vi "calibration.vi"() -> ()   [LabVIEW 2012]
uses:
  globalstatus.vi
  globalreport.vi
  globalsettings.vi
panel:
  in  "in sn 3":string
  in  "status":u16(ring) items=["idle", "read sn", "write sn", "adjust dac", "collect", "write coefficient", "check do"]
  in  "in sn 7":string
  out "working 7":bool
  out "sn 7":string
  in  "port 7":refnum<visa-resource-name>
  in  "in sn 6":string
  out "working 6":bool
  out "sn 6":string
  in  "port 6":refnum<visa-resource-name>
  in  "in sn 5":string
  out "working 5":bool
  out "sn 5":string
  in  "port 5":refnum<visa-resource-name>
  in  "in sn 4":string
  out "working 4":bool
  out "sn 4":string
  in  "port 4":refnum<visa-resource-name>
  out "working 3":bool
  out "sn 3":string
  in  "port 3":refnum<visa-resource-name>
  in  "in sn 2":string
  in  "in sn 1":string
  out "working 2":bool
  out "working 1":bool
  out "working":bool
  out "sn 2":string
  out "sn 1":string
  out "sn":string
  in  "run":bool
  in  "golden port":refnum<visa-resource-name>
  in  "port 2":refnum<visa-resource-name>
  in  "port 1":refnum<visa-resource-name>
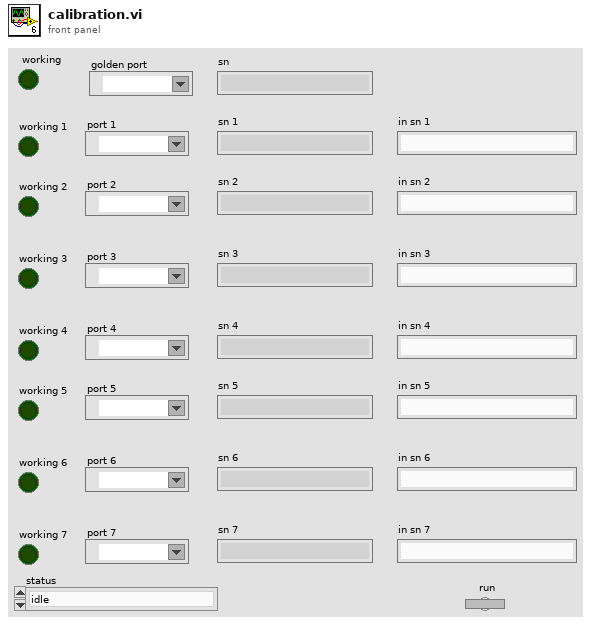
[diagram p1: front panel]
types:
  T1 = cluster{"B0":dbl, "B1":dbl, "K":dbl, "B":dbl, "B2":dbl}
  T2 = cluster{"port 7":refnum<visa-resource-name>, string, dbl, dbl, dbl, dbl, dbl, dbl, dbl, dbl, dbl, dbl, dbl, dbl, dbl, dbl, dbl, "B0":dbl, "B1":dbl, "B2":dbl, "K":dbl, "B":dbl, string, string}
  T3 = cluster{"Ten 0%":dbl, "Ten 5%":dbl, "Ten 10%":dbl, "Ten 20%":dbl, "Tolerance":dbl, "Ten 15%":dbl, "Ten 40%":dbl, "Ten 100%":dbl, "Times":dbl}
  T4 = cluster{"PORT":string, "SN":string, "RED DAC":dbl, "BLUE DAC":dbl, "RED AMP":dbl, "BLUE AMP":dbl, "T0":dbl, "T1":dbl, "T2":dbl, "T3":dbl, "T4":dbl, "T5":dbl, "T6":dbl, "A0":dbl, "A1":dbl, "A2":dbl, "A3":dbl, "B0":dbl, "B1":dbl, "B2":dbl, "C1":dbl, "C0":dbl, "result":string, "error":string}[]
  T5 = cluster{"port 7":refnum<visa-resource-name>, string, string, string, string, string, string, string, string, string, string}
  T6 = cluster{"DO 0%":dbl, "DO 5%":dbl, "DO 10%":dbl, "DO 20%":dbl, "Tolerance":dbl, "DO 15%":dbl, "DO 40%":dbl, "DO 100%":dbl, "Times":dbl}
  T7 = cluster{"PORT":string, "SN":string, "DO 0":string, "DO 1":string, "DO 2":string, "DO 3":string, "DO 4":string, "DO 5":string, "DO 6":string, "result":string, "error":string}[]
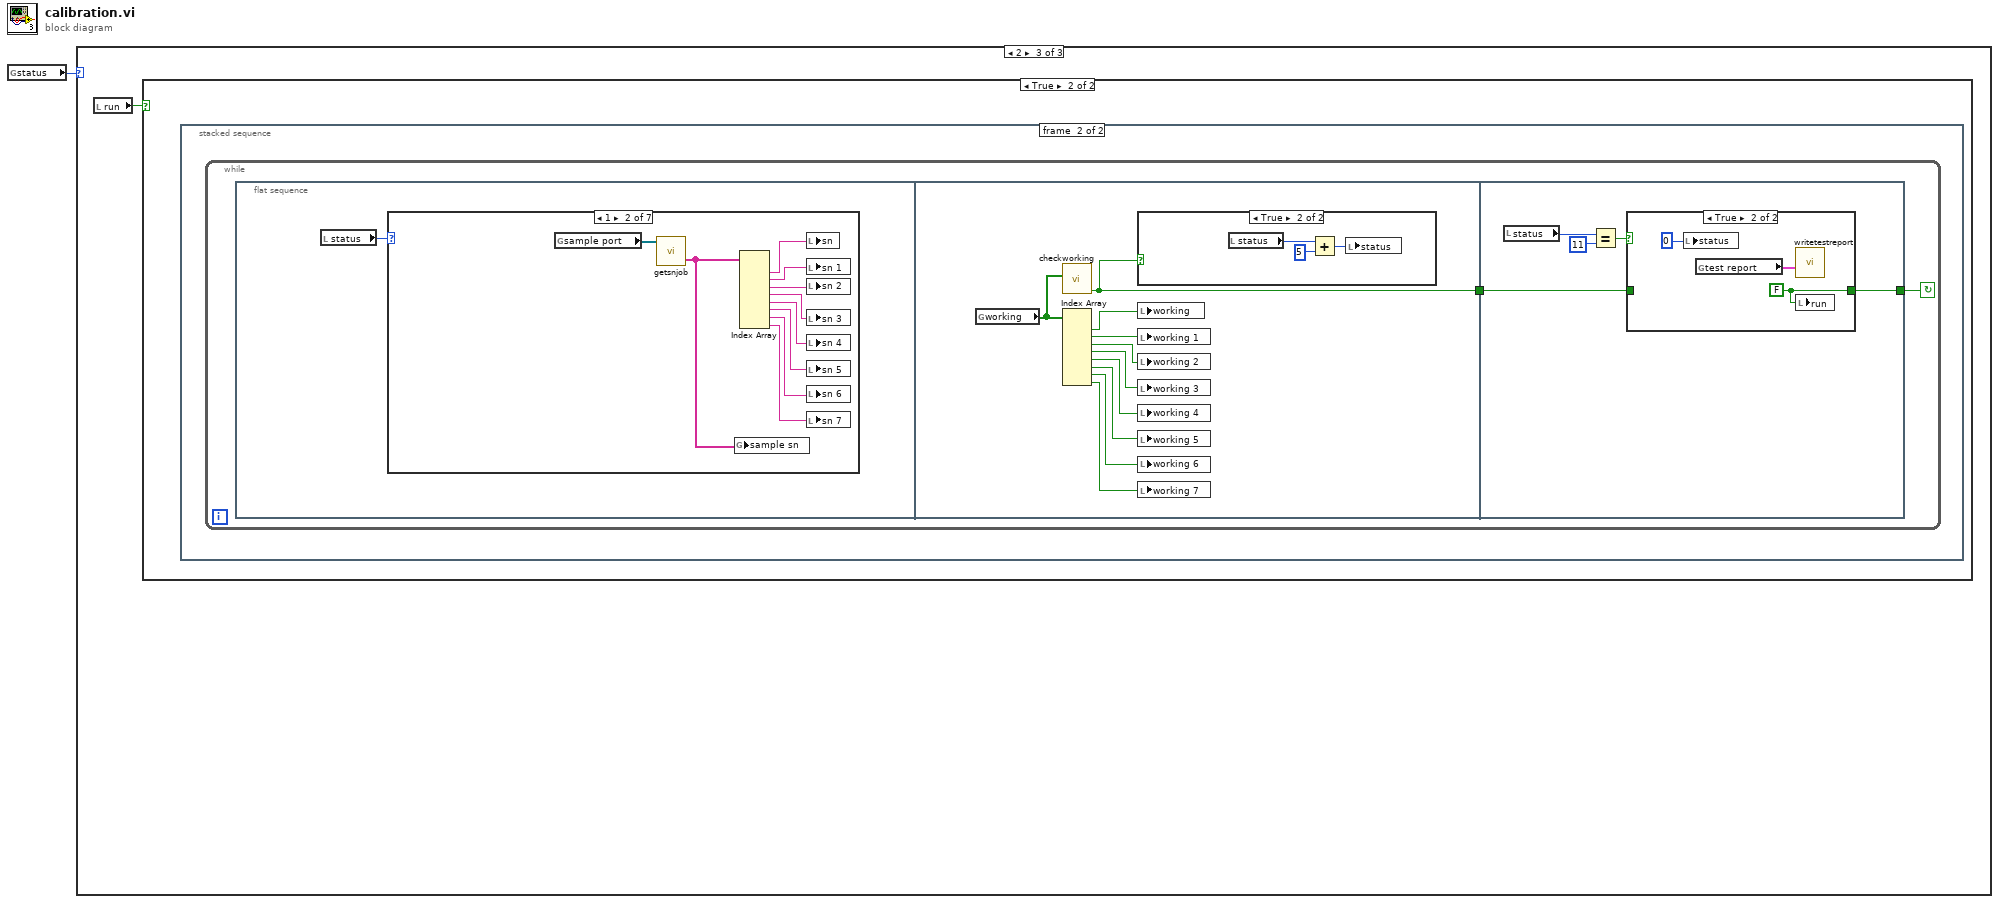
[diagram p0: block diagram]
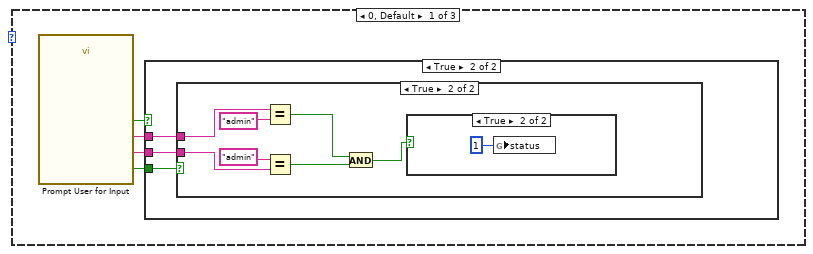
[diagram p2: hidden frame]
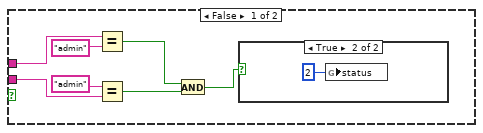
[diagram p4: hidden frame]
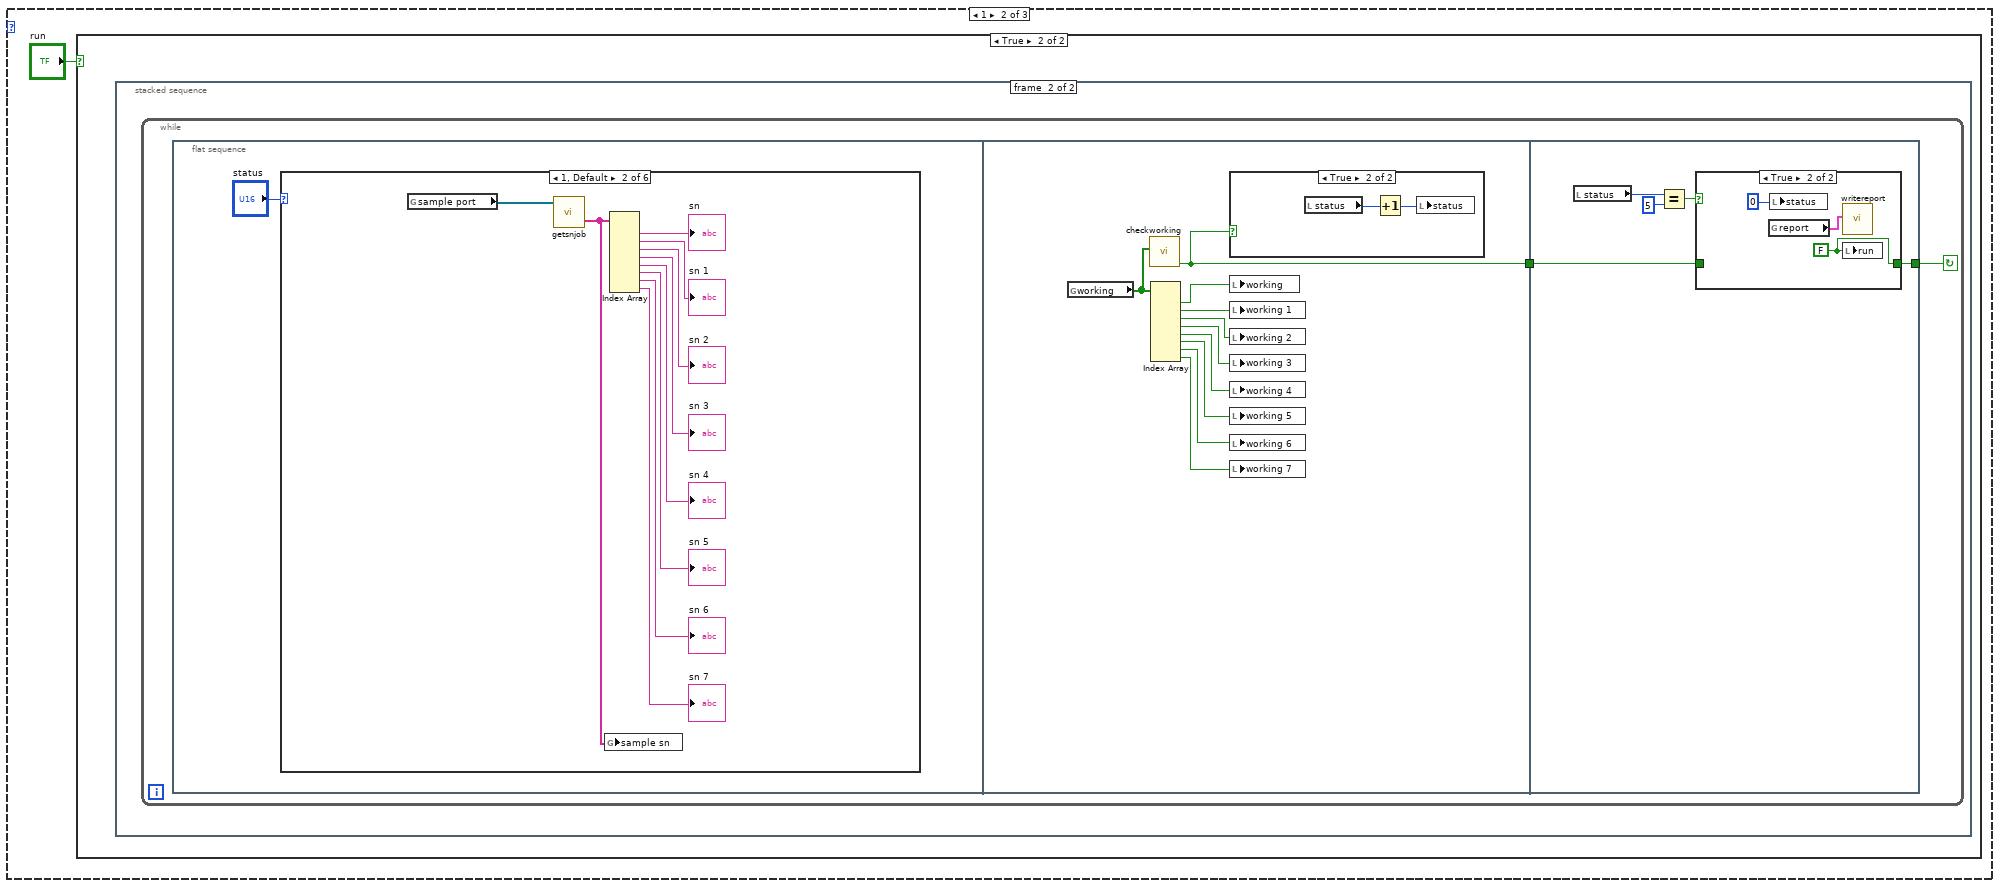
[diagram p7: hidden frame]
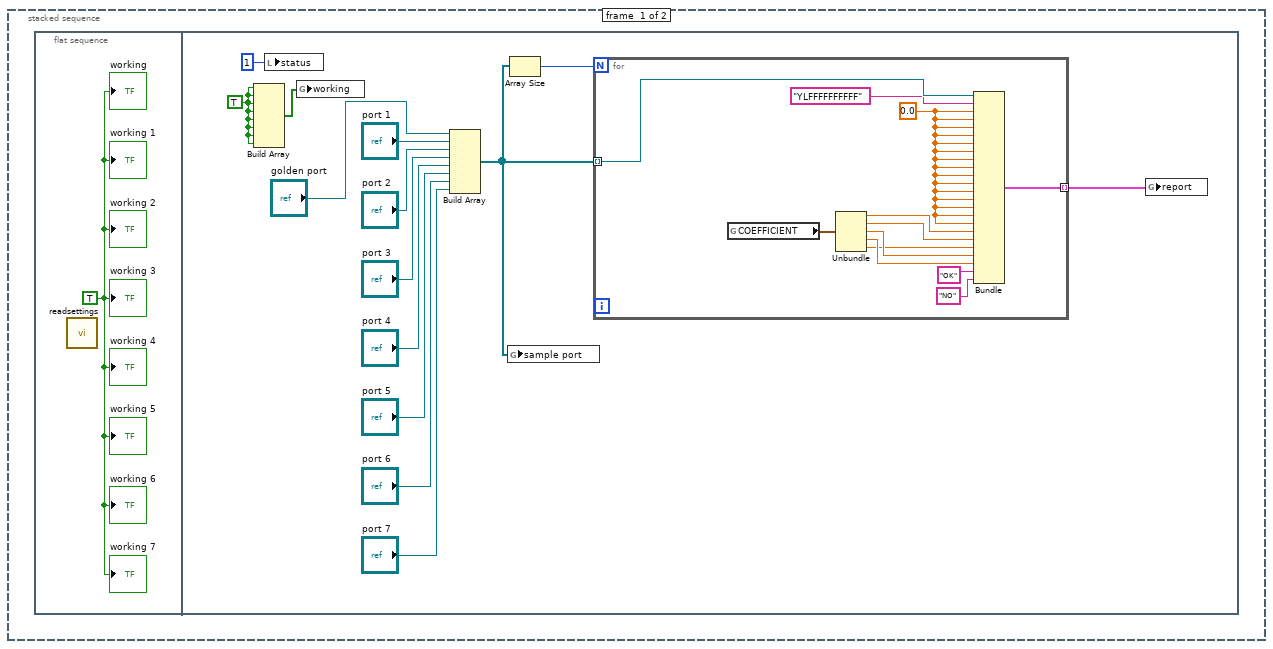
[diagram p9: hidden frame]
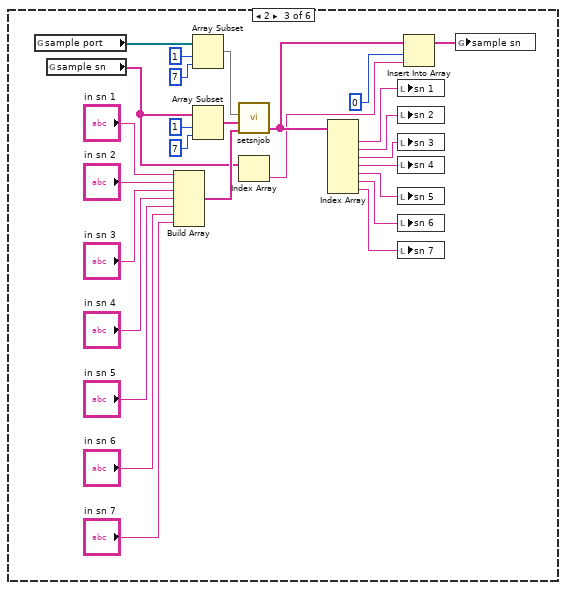
[diagram p11: hidden frame]
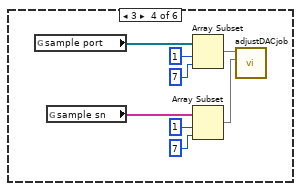
[diagram p12: hidden frame]
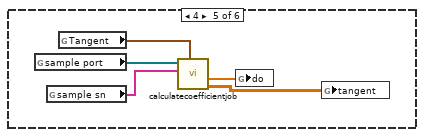
[diagram p13: hidden frame]
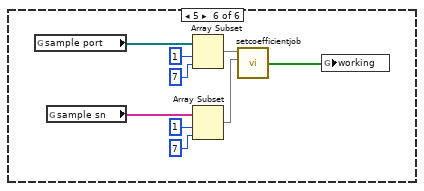
[diagram p14: hidden frame]
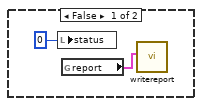
[diagram p15: hidden frame]
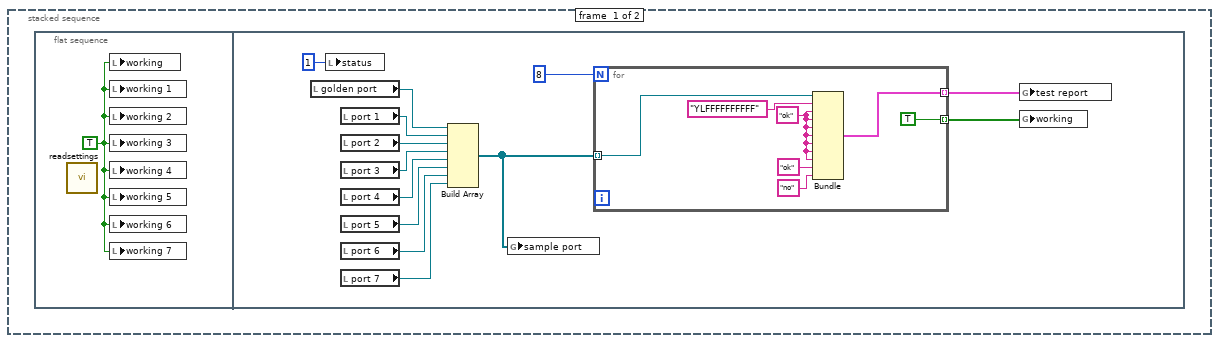
[diagram p18: hidden frame]
diagram:
  n1 = global read "globalstatus.vi" "status"() -> (w1:u16)
  n2 = case shown="2" w1 {
    frame 0, Default {
      n3 = call "Prompt User for Input"() -> ("calibrate"=w4:bool, "password"=w3:string, "name"=w2:string, "OK"=w5:bool)  [unwired: 15 in, 1 out]
      n4 = case shown="True" w5 {
        tunnel: w4 -> [_ w8]
        tunnel: w3 -> [_ w7]
        tunnel: w2 -> [_ w6]
        frame False {
        }
        frame True {
          n5 = case shown="True" w8 {
            tunnel: w7 -> [w11 w19]
            tunnel: w6 -> [w12 w18]
            frame False {
              n6 = Equal?(x=w12, y="admin") -> (x = y?=w15:bool)
              n7 = Equal?(x="admin", y=w11) -> (x = y?=w10:bool)
              n8 = And(x=w15, y=w10) -> (x .and. y?=w9:bool)
              n9 = case shown="True" w9 {
                frame False {
                }
                frame True {
                  n10 = global write "globalstatus.vi" "status"(2) -> ()
                }
              }
            }
            frame True {
              n11 = Equal?(x=w18, y="admin") -> (x = y?=w22:bool)
              n12 = Equal?(x="admin", y=w19) -> (x = y?=w23:bool)
              n13 = And(x=w22, y=w23) -> (x .and. y?=w17:bool)
              n14 = case shown="True" w17 {
                frame False {
                }
                frame True {
                  n15 = global write "globalstatus.vi" "status"(1) -> ()
                }
              }
            }
          }
        }
      }
    }
    frame 1 {
      n16 = case shown="True" "run" {
        frame False {
        }
        frame True {
          n17 = stacked-sequence {
            frame #0 {
              n18 = flat-sequence {
                frame #0 {
                  w26 = TRUE
                  n19 = call "readsettings.vi"() -> ()  [unwired: 11 in, 1 out]
                  "working" <- w26
                  "working 1" <- w26
                  "working 2" <- w26
                  "working 7" <- w26
                  "working 6" <- w26
                  "working 5" <- w26
                  "working 4" <- w26
                  "working 3" <- w26
                }
                frame #1 {
                  w37 = TRUE
                  n20 = Build Array(w37, w37, w37, w37, w37, w37, w37, w37) -> (w38:bool[])
                  n21 = local write "status"(1) -> ()
                  n22 = global write "globalstatus.vi" "working"(w38) -> ()
                  n23 = Build Array("golden port", "port 1", "port 2", "port 3", "port 4", "port 5", "port 6", "port 7") -> (w28:refnum<visa-resource-name>[])
                  n24 = global write "globalstatus.vi" "sample port"(w28) -> ()
                  n25 = Array Size(array=w28) -> (size(s)=w39:i32)
                  n26 = for {
                    N: w39 -> [_]
                    tunnel: [w46] -> w40 mode=indexing
                    tunnel: w28 -> [w45] mode=indexing
                    w41 = 0.0
                    n27 = global read "globalsettings.vi" "COEFFICIENT"() -> (w52:T1)
                    n28 = Unbundle(w52) -> ("B0"=w51:dbl, "B1"=w50:dbl, "K"=w49:dbl, "B"=w48:dbl, "B2"=w47:dbl)
                    n29 = Bundle("port 7"=w45, "YLFFFFFFFFFF", w41, w41, w41, w41, w41, w41, w41, w41, w41, w41, w41, w41, w41, w41, w41, "B0"=w51, "B1"=w50, "B2"=w47, "K"=w49, "B"=w48, "OK", "NO") -> (w46:T2)  [unwired: 1 in]
                  }
                  n30 = global write "globalreport.vi" "report"(w40) -> ()
                }
              }
            }
            frame #1 {
              n31 = while {
                stop <- w54 continue-if-true
                n32 = flat-sequence {
                  tunnel: [w124] -> w53
                  tunnel: [w129] -> w54
                  tunnel: w53 -> [w130]
                  frame #0 {
                    n33 = case shown="1, Default" "status" {
                      frame 0 {
                      }
                      frame 1, Default {
                        n34 = global read "globalstatus.vi" "sample port"() -> (w57:refnum<visa-resource-name>[])
                        n35 = call "getsnjob.vi"("sample port"=w57) -> ("sample sn"=w56:string[])  [unwired: 3 in]
                        n36 = global write "globalstatus.vi" "sample sn"(w56) -> ()
                        n37 = Index Array(array=w56) -> (element #1=→"sn":string, element #2=→"sn 1":string, element #3=→"sn 2":string, element #4=→"sn 3":string, element #5=→"sn 4":string, element #6=→"sn 5":string, element #7=→"sn 6":string, element #8=→"sn 7":string)  [unwired: 8 in]
                      }
                      frame 2 {
                        n38 = global read "globalstatus.vi" "sample port"() -> (w78:refnum<visa-resource-name>[])
                        n39 = global read "globalstatus.vi" "sample sn"() -> (w73:string[])
                        n40 = Build Array("in sn 1", "in sn 2", "in sn 3", "in sn 4", "in sn 5", "in sn 6", "in sn 7") -> (w92:string[])
                        n41 = Array Subset(array=w78, index=1, length=7) -> (w82:refnum<visa-resource-name>[])
                        n42 = Array Subset(array=w73, index=1, length=7) -> (w81:string[])
                        n43 = call "setsnjob.vi"("sample sn"=w92, "sample old sn"=w81, "sample port"=w82) -> ("sample sn out"=w77:string[])  [unwired: 3 in]
                        n44 = Index Array(array=w73) -> (element=w76:string)  [unwired: 1 in]
                        n45 = Index Array(array=w77) -> (element #1=w91:string, element #2=w90:string, element #3=w89:string, element #4=w88:string, element #5=w87:string, element #6=w86:string, element #7=w85:string)  [unwired: 7 in]
                        n46 = local write "sn 1"(w91) -> ()
                        n47 = local write "sn 2"(w90) -> ()
                        n48 = local write "sn 3"(w89) -> ()
                        n49 = local write "sn 4"(w88) -> ()
                        n50 = local write "sn 5"(w87) -> ()
                        n51 = local write "sn 6"(w86) -> ()
                        n52 = local write "sn 7"(w85) -> ()
                        n53 = Insert Into Array(array=w77, index=0, new element=w76) -> (w74:string[])
                        n54 = global write "globalstatus.vi" "sample sn"(w74) -> ()
                      }
                      frame 3 {
                        n55 = global read "globalstatus.vi" "sample port"() -> (w94:refnum<visa-resource-name>[])
                        n56 = global read "globalstatus.vi" "sample sn"() -> (w93:string[])
                        n57 = Array Subset(array=w94, index=1, length=7) -> (w95:refnum<visa-resource-name>[])
                        n58 = Array Subset(array=w93, index=1, length=7) -> (w96:string[])
                        n59 = call "adjustDACjob.vi"("sample sn"=w96, "sample port"=w95) -> ()  [unwired: 10 in]
                      }
                      frame 4 {
                        n60 = global read "globalstatus.vi" "sample port"() -> (w102:refnum<visa-resource-name>[])
                        n61 = global read "globalstatus.vi" "sample sn"() -> (w101:string[])
                        n62 = global read "globalsettings.vi" "Tangent"() -> (w103:T3)
                        n63 = call "calculatecoefficientjob.vi"("Tangent"=w103, "sample sn"=w101, "sample port"=w102) -> ("tangent"=w104:dbl[][], "do"=w105:dbl[])  [unwired: 7 in]
                        n64 = global write "globalstatus.vi" "do"(w105) -> ()
                        n65 = global write "globalstatus.vi" "tangent"(w104) -> ()
                      }
                      frame 5 {
                        n66 = global read "globalstatus.vi" "sample port"() -> (w108:refnum<visa-resource-name>[])
                        n67 = global read "globalstatus.vi" "sample sn"() -> (w107:string[])
                        n68 = Array Subset(array=w108, index=1, length=7) -> (w110:refnum<visa-resource-name>[])
                        n69 = Array Subset(array=w107, index=1, length=7) -> (w109:string[])
                        n70 = call "setcoefficientjob.vi"("sample port"=w110, "sample sn"=w109) -> ("Array"=w106:bool[])  [unwired: 6 in]
                        n71 = global write "globalstatus.vi" "working"(w106) -> ()
                      }
                    }
                  }
                  frame #1 {
                    n72 = global read "globalstatus.vi" "working"() -> (w115:bool[])
                    n73 = call "checkworking.vi"("Array"=w115) -> ("Boolean"=w124:bool)  [unwired: 8 in]
                    n74 = Index Array(array=w115) -> (element #1=w123:bool, element #2=w122:bool, element #3=w121:bool, element #4=w120:bool, element #5=w119:bool, element #6=w118:bool, element #7=w117:bool, element #8=w116:bool)  [unwired: 8 in]
                    n75 = case shown="True" w124 {
                      frame False {
                        n76 = local write "status"(0) -> ()
                        n77 = global read "globalreport.vi" "report"() -> (w125:T4)
                        n78 = call "writereport.vi"("Array"=w125) -> ()  [unwired: 11 in]
                      }
                      frame True {
                        n79 = local read "status"() -> (w128:u16)
                        n80 = Increment(x=w128) -> (x+1=w127:u16)
                        n81 = local write "status"(w127) -> ()
                      }
                    }
                    n82 = local write "working"(w123) -> ()
                    n83 = local write "working 1"(w122) -> ()
                    n84 = local write "working 2"(w121) -> ()
                    n85 = local write "working 3"(w120) -> ()
                    n86 = local write "working 4"(w119) -> ()
                    n87 = local write "working 5"(w118) -> ()
                    n88 = local write "working 6"(w117) -> ()
                    n89 = local write "working 7"(w116) -> ()
                  }
                  frame #2 {
                    n90 = local read "status"() -> (w133:u16)
                    n91 = Equal?(x=w133, y=5) -> (x = y?=w131:bool)
                    n92 = case shown="True" w131 {
                      tunnel: w130 -> [w134 _]
                      tunnel: [w134 w137] -> w129
                      frame False {
                      }
                      frame True {
                        w137 = FALSE
                        n93 = global read "globalreport.vi" "report"() -> (w135:T4)
                        n94 = local write "status"(0) -> ()
                        n95 = call "writereport.vi"("Array"=w135) -> ()  [unwired: 11 in]
                        n96 = local write "run"(w137) -> ()
                      }
                    }
                  }
                }
              }
            }
          }
        }
      }
    }
    frame 2 {
      n97 = local read "run"() -> (w138:bool)
      n98 = case shown="True" w138 {
        frame False {
        }
        frame True {
          n99 = stacked-sequence {
            frame #0 {
              n100 = flat-sequence {
                frame #0 {
                  w139 = TRUE
                  n101 = call "readsettings.vi"() -> ()  [unwired: 11 in, 1 out]
                  n102 = local write "working"(w139) -> ()
                  n103 = local write "working 1"(w139) -> ()
                  n104 = local write "working 2"(w139) -> ()
                  n105 = local write "working 3"(w139) -> ()
                  n106 = local write "working 4"(w139) -> ()
                  n107 = local write "working 5"(w139) -> ()
                  n108 = local write "working 6"(w139) -> ()
                  n109 = local write "working 7"(w139) -> ()
                }
                frame #1 {
                  n110 = local read "golden port"() -> (w143:refnum<visa-resource-name>)
                  n111 = local write "status"(1) -> ()
                  n112 = local read "port 1"() -> (w144:refnum<visa-resource-name>)
                  n113 = local read "port 2"() -> (w145:refnum<visa-resource-name>)
                  n114 = local read "port 3"() -> (w146:refnum<visa-resource-name>)
                  n115 = local read "port 4"() -> (w147:refnum<visa-resource-name>)
                  n116 = local read "port 5"() -> (w148:refnum<visa-resource-name>)
                  n117 = local read "port 6"() -> (w149:refnum<visa-resource-name>)
                  n118 = local read "port 7"() -> (w150:refnum<visa-resource-name>)
                  n119 = Build Array(w143, w144, w145, w146, w147, w148, w149, w150) -> (w140:refnum<visa-resource-name>[])
                  n120 = global write "globalstatus.vi" "sample port"(w140) -> ()
                  n121 = for {
                    N: 8 -> [_]
                    tunnel: [TRUE] -> w151 mode=indexing
                    tunnel: [w158] -> w141 mode=indexing
                    tunnel: w140 -> [w157] mode=indexing
                    w153 = "ok"
                    n122 = Bundle("port 7"=w157, "YLFFFFFFFFFF", w153, w153, w153, w153, w153, w153, w153, "ok", "no") -> (w158:T5)  [unwired: 1 in]
                  }
                  n123 = global write "globalreport.vi" "test report"(w141) -> ()
                  n124 = global write "globalstatus.vi" "working"(w151) -> ()
                }
              }
            }
            frame #1 {
              n125 = while {
                stop <- w160 continue-if-true
                n126 = flat-sequence {
                  tunnel: [w176] -> w161
                  tunnel: [w190] -> w160
                  tunnel: w161 -> [w189]
                  frame #0 {
                    n127 = local read "status"() -> (w162:u16)
                    n128 = case shown="1" w162 {
                      frame 0, Default {
                      }
                      frame 1 {
                        n129 = global read "globalstatus.vi" "sample port"() -> (w172:refnum<visa-resource-name>[])
                        n130 = call "getsnjob.vi"("sample port"=w172) -> ("sample sn"=w171:string[])  [unwired: 3 in]
                        n131 = global write "globalstatus.vi" "sample sn"(w171) -> ()
                        n132 = Index Array(array=w171) -> (element #1=w163:string, element #2=w164:string, element #3=w165:string, element #4=w166:string, element #5=w167:string, element #6=w168:string, element #7=w169:string, element #8=w170:string)  [unwired: 8 in]
                        n133 = local write "sn"(w163) -> ()
                        n134 = local write "sn 1"(w164) -> ()
                        n135 = local write "sn 2"(w165) -> ()
                        n136 = local write "sn 3"(w166) -> ()
                        n137 = local write "sn 4"(w167) -> ()
                        n138 = local write "sn 5"(w168) -> ()
                        n139 = local write "sn 6"(w169) -> ()
                        n140 = local write "sn 7"(w170) -> ()
                      }
                      frame 2 {
                      }
                      frame 3 {
                      }
                      frame 4 {
                      }
                      frame 5 {
                      }
                      frame 6 {
                        n141 = global read "globalstatus.vi" "sample sn"() -> (w175:string[])
                        n142 = global read "globalstatus.vi" "sample port"() -> (w174:refnum<visa-resource-name>[])
                        n143 = global read "globalsettings.vi" "DO"() -> (w173:T6)
                        n144 = call "checkdojob.vi"("DO"=w173, "sample sn"=w175, "sample port"=w174) -> ()  [unwired: 8 in, 1 out]
                      }
                    }
                  }
                  frame #1 {
                    n145 = global read "globalstatus.vi" "working"() -> (w185:bool[])
                    n146 = call "checkworking.vi"("Array"=w185) -> ("Boolean"=w176:bool)  [unwired: 8 in]
                    n147 = Index Array(array=w185) -> (element #1=w184:bool, element #2=w183:bool, element #3=w182:bool, element #4=w181:bool, element #5=w180:bool, element #6=w179:bool, element #7=w178:bool, element #8=w177:bool)  [unwired: 8 in]
                    n148 = case shown="True" w176 {
                      frame False {
                      }
                      frame True {
                        n149 = local read "status"() -> (w188:u16)
                        n150 = Add(x=w188, y=5) -> (x+y=w186:i32)
                        n151 = local write "status"(w186) -> ()
                      }
                    }
                    n152 = local write "working"(w184) -> ()
                    n153 = local write "working 1"(w183) -> ()
                    n154 = local write "working 2"(w182) -> ()
                    n155 = local write "working 3"(w181) -> ()
                    n156 = local write "working 4"(w180) -> ()
                    n157 = local write "working 5"(w179) -> ()
                    n158 = local write "working 6"(w178) -> ()
                    n159 = local write "working 7"(w177) -> ()
                  }
                  frame #2 {
                    n160 = local read "status"() -> (w192:u16)
                    n161 = Equal?(x=w192, y=11) -> (x = y?=w191:bool)
                    n162 = case shown="True" w191 {
                      tunnel: [w194 w197] -> w190
                      tunnel: w189 -> [w194 _]
                      frame False {
                      }
                      frame True {
                        w197 = FALSE
                        n163 = local write "status"(0) -> ()
                        n164 = global read "globalreport.vi" "test report"() -> (w195:T7)
                        n165 = call "writetestreport.vi"("test report"=w195) -> ()  [unwired: 11 in]
                        n166 = local write "run"(w197) -> ()
                      }
                    }
                  }
                }
              }
            }
          }
        }
      }
    }
  }
